vi "Add FIU Card.vi"(8 "error in (no error)":errorcluster, 11 "Node Ptr":u64 format="%.0x") -> (0 "error out":errorcluster)   [LabVIEW 2014, in "SLSC configuration System Explorer.lvlib"]
uses:
  SLSC configuration System Explorer.lvlib
  Shared/Constants.vi
  Shared/SLSC configuration Shared.lvlib
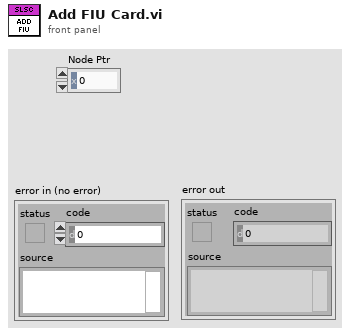
[diagram p1: front panel]
types:
  T1 = typedef "SLSC configuration Shared.lvlib/Card Position.ctl" = cluster{"Rack #":u8, "Slot #":T2}
  T2 = typedef "SLSC configuration Shared.lvlib/Slot #.ctl" = u8
  T3 = typedef "Custom Device API.lvlib/Custom Device Item Ref.ctl" = u64
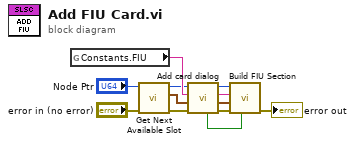
[diagram p0: block diagram]
diagram:
  n1 = global read "Constants.vi" "Constants.FIU"() -> (w8:string)
  n2 = call "Get Next Available Slot.vi"("error in (no error)"="error in (no error)", "Device Ref in"="Node Ptr") -> ("error out"=w4:errorcluster, "Next Open Slot"=w3:T1, "Device Ref out"=w1:T3)  [unwired: 7 in]
  n3 = call "Add card dialog.vi"("error in (no error)"=w4, "Card Position"=w3, "Card Type in"=w8, "Node Ptr"=w1) -> ("error out"=w10:errorcluster, "Card Position out"=w9:T1, "Name out"=w11:string, "Node Ptr out"=w12:u64, "Cancelled?"=w6:bool)  [unwired: 3 in]
  n4 = call "Build FIU Section.vi"("Cancelled?"=w6, "error in (no error)"=w10, "Card Position in"=w9, "Name in"=w11, "Node Ptr in"=w12) -> ("error out"=→"error out":errorcluster)  [unwired: 6 in]
